vi "按钮旋转.vi"() -> ()   [LabVIEW 2018]
panel:
  out "布尔 4":bool
  out "布尔 3":bool
  out "布尔 2":bool
  in  "确定按钮":bool
  in  "停止":bool
  out "布尔":bool
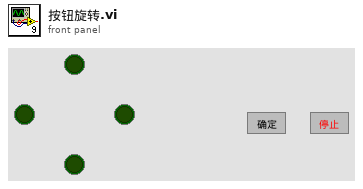
[diagram p1: front panel]
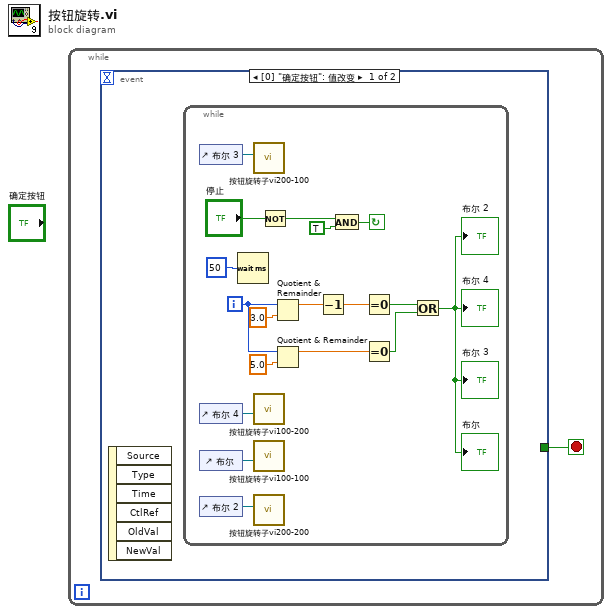
[diagram p0: block diagram]
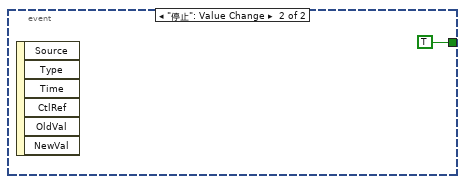
[diagram p2: hidden frame]
diagram:
  n1 = while {
    stop <- w1 stop-if-true
    n2 = event shown="[0] \"确定按钮\": 值改变" {
      selector: _ -> [_ _]
      dyn-events: _ -> [_ _]
      timeout: _ -> [_ _]
      tunnel: [_ TRUE] -> w1
      event "确定按钮": Value Change {
        n3 = event-data() -> ()  [unwired: 1 in, 6 out]
        n4 = while {
          i -> [w12]
          stop <- w4 continue-if-true
          n5 = control-ref of="布尔 3"() -> (w18:refnum<vi>)
          n6 = control-ref of="布尔 4"() -> (w19:refnum<vi>)
          n7 = control-ref of="布尔"() -> (w6:refnum<vi>)
          n8 = control-ref of="布尔 2"() -> (w17:refnum<vi>)
          n9 = Wait (ms)(milliseconds to wait=u32 50 ("等待时间（毫秒）")) -> ()  [unwired: 1 out]
          n10 = call "按钮旋转子vi200-100.vi"("Ctl引用句柄"=w18) -> ()  [unwired: 11 in]
          n11 = call "按钮旋转子vi100-200.vi"("Ctl引用句柄"=w19) -> ()  [unwired: 11 in]
          n12 = call "按钮旋转子vi100-100.vi"("Ctl引用句柄"=w6) -> ()  [unwired: 10 in]
          n13 = call "按钮旋转子vi200-200.vi"("Ctl引用句柄"=w17) -> ()  [unwired: 11 in]
          n14 = Not(x="停止") -> (.not. x?=w2:bool)
          n15 = Quotient & Remainder(x=w12, y=3.0) -> (x-y*floor(x/y)=w11:dbl)  [unwired: 1 out]
          n16 = Quotient & Remainder(x=w12, y=5.0) -> (x-y*floor(x/y)=w15:dbl)  [unwired: 1 out]
          n17 = Decrement(x=w11) -> (x-1=w10:dbl)
          n18 = And(x=w2, y=TRUE) -> (x .and. y?=w4:bool)
          n19 = Equal To 0?(x=w10) -> (x = 0?=w9:bool)
          n20 = Equal To 0?(x=w15) -> (x = 0?=w8:bool)
          n21 = Or(x=w9, y=w8) -> (x .or. y?=→"布尔 2" →"布尔 4" →"布尔 3" →"布尔":bool)
        }
      }
      event "停止": Value Change {
        n22 = event-data() -> ()  [unwired: 1 in, 6 out]
      }
    }
  }
